vi "Is Command.vi"(6 "Level":T1, 7 "Message":refnum<class "Message Interface.lvclass">, 8 "error in (no error)":errorcluster, 11 "Mediated Actor in":refnum<class "Mediated Actor.lvclass">) -> (0 "error out":errorcluster, 1 "Command Message?":bool, 2 "Command Name":string, 3 "Mediated Actor out":refnum<class "Mediated Actor.lvclass">)   [LabVIEW 2016, in "Stream Mediator.lvlib" / "Mediated Actor.lvclass"]
doc: "--\nCopyright © 2017 Composed SystemsI All rights reserved.\n\nAuthor: Jon McBee <jon.mcbee@composed.io>\n\nThis library is provided \"AS IS\" ,WITHOUT WARRANTIES OR\nCONDITIONS OF ANY KIND, either express or implied.\n\nComposed Systems -- composed.io\n\nStream 0.0.1.1\nJon McBee - Composed Systems\nCopyright (c) 2017, Composed Systems"
uses:
  <userlib>/Composed Systems/Stream/Mediator/Classes/Mediated Actor/Mediated Actor.lvclass
  C:/Program Files (x86)/National Instruments/LabVIEW 2016/user.lib/Composed Systems/Stream/Actor/Actor Class/Ancestral Actor.lvclass
  <userlib>/Composed Systems/Stream/Log/Application Log/Log Level.ctl
  <userlib>/Composed Systems/Stream/Mediator/Classes/Message Interface/Message Interface.lvclass
  <userlib>/Composed Systems/Stream/Mediator/Classes/Message Command Interface/Command Message Interface.lvclass
  C:/Program Files (x86)/National Instruments/LabVIEW 2016/user.lib/Composed Systems/Stream/Mediator/Classes/Message Interface/Message Interface.lvclass
  <userlib>/Composed Systems/Stream/Log/Global Application Log/Global Application Log.lvclass
  <userlib>/Composed Systems/Stream/Log/Application Log/Application Log.lvclass
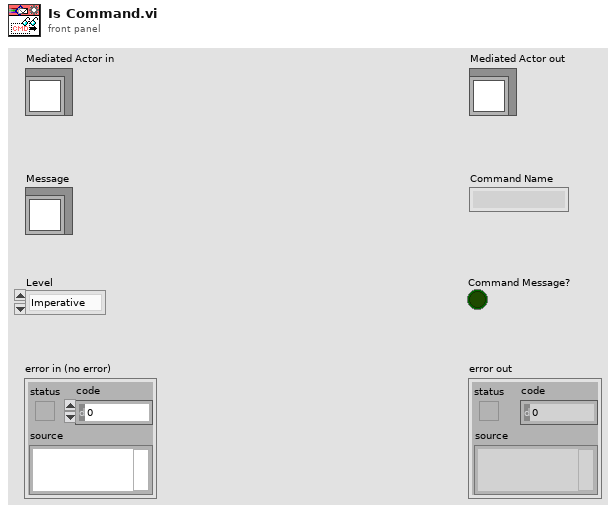
[diagram p1: front panel]
types:
  T1 = typedef "Stream Log.lvlib/Application Log.lvclass/Log Level.ctl" = enum16{"Imperative", "Major", "Minor", "Debug", "Off"}
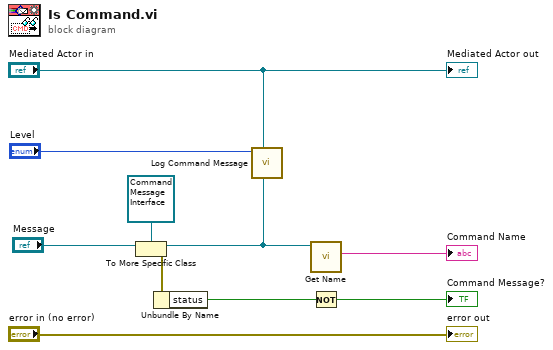
[diagram p0: block diagram]
diagram:
  n1 = To More Specific Class(target class=refnum<class "Command Message Interface.lvclass"> refnum ("Mediator Framework.lvlib:Command Message Interface.lvclass"), reference="Message") -> (specific class reference=w5:refnum<class "Command Message Interface.lvclass">, error out=w4:errorcluster)  [unwired: 1 in]
  n2 = Unbundle By Name(w4) -> ("status"=w3:bool)
  n3 = call <userlib>:"Log Command Message.vi"("Command Message"=w5, "Actor"="Mediated Actor in", "Level"="Level") -> ()  [unwired: 8 in, 1 out]
  n4 = call <userlib>:"Get Name.vi"("Message Interface in"=w5) -> ("Name"=→"Command Name":string)  [unwired: 8 in, 2 out]
  n5 = Not(x=w3) -> (.not. x?=→"Command Message?":bool)
  "error out" <- "error in (no error)"
  "Mediated Actor out" <- "Mediated Actor in"
